vi "Home Page.vi"() -> (4 "Home Msg":string="    Parameters for measuring ADC: \n\n            1. DNL  \n\n            2. INL  \n\n \nDNL:\n\n   * Differential Non-Linearity (DNL) is the difference between two successive voltage levels that the DAC produces. \n\n   * Difference between the actual step width occurred and ideal step width for the corresponding voltage. \n\n   * The ideal difference between two successive voltages is 1 LSB. \n\n   * To generate DNL, take the difference of  Vout value from one transition to the next transition and ideal value. \n\nINL:\n\n   * Integral Non-Linearity (INL) is the maximum deviation of actual input-output characteristics from the ideal transfer characteristics. \n\n   * It is measured by using the Endpoint method. \n\n   * If the INL of a DAC is less than ±0.5 LSb, the input-output characteristic is monotonic.  ")   [LabVIEW 2020, in "INL DNL Test.lvclass"]
doc: "Home page to display the information about the test."
uses:
  INL DNL Test.lvclass
  Typedef/User event controls.ctl
  DNL INL Test.lvlib
panel:
  out "Error Out":errorcluster
  in  "Error In":errorcluster
  # "DNL and INL Test"
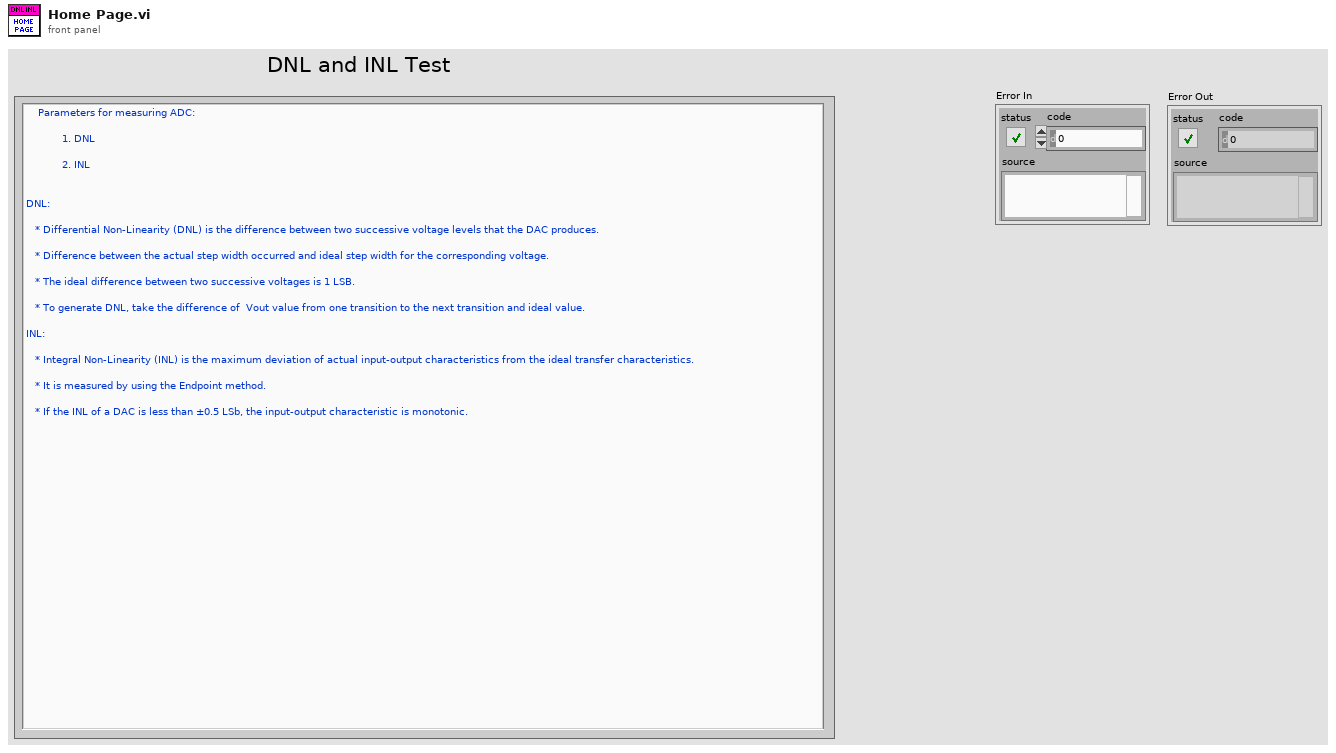
[diagram p1: front panel]
types:
  T1 = typedef "DNL INL Test.lvlib/User event controls.ctl" = enum16{"Create", "Generate", "Run Test", "Get Ref", "Destroy"}
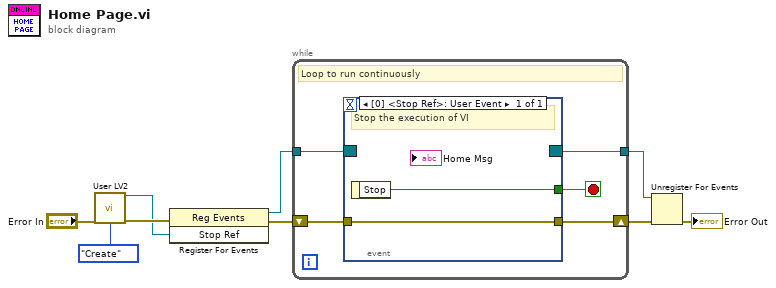
[diagram p0: block diagram]
diagram:
  n1 = call "User LV2.vi"("Error In"="Error In", "User event controls"=User_event_controls."Create") -> ("Stop Ref"=w5:refnum<user-event>, "Error Out"=w7:errorcluster)  [unwired: 11 in, 1 out]
  n2 = register-events(error in=w7, w5) -> (reference out=w9:refnum<event-registration>, error out=w4:errorcluster)  [unwired: 1 in]
  n3 = while {
    tunnel: w9 -> [w14]
    tunnel: [w12] -> w2
    shift-right: [w10] -> w3
    shift-left: w4 -> [w11]
    stop <- w13 stop-if-true
    # "Loop to run continuously"
    n4 = event shown="[0] <Stop Ref>: User Event" {
      selector: w14 -> [_]
      dyn-events: [_] -> w12
      timeout: _ -> [_]
      tunnel: [w16] -> w13
      tunnel: [w15] -> w10
      tunnel: w11 -> [w15]
      event User Event {
        # "Stop the execution of VI"
        n5 = event-data() -> ("Stop"=w16:bool)  [unwired: 1 in]
      }
    }
  }
  n6 = Unregister For Events(event registration refnum=w2, error in=w3) -> (error out=→"Error Out":errorcluster)
